vi "RSZVB Get IMOD Upper Tone Source.vi"(8 "error in (no error)":errorcluster {"code" format="%.0x"}, 10 "Channel (1)":i32=1, 11 "VISA session":refnum<visa-resource-name>) -> (0 "error out":errorcluster {"code" format="%.0x"}, 1 "Source":i32, 3 "dup VISA session":refnum<visa-resource-name>, 5 "Source Number":i32)   [LabVIEW 2011]
doc: "This VI returns the source for the upper tone signal that is used for the intermodulation measurement.\n\nNote(s):\n\n(1) This VI is not available for R&S ZVB instrument.\n\nRemote-control command(s):\n[SENSe<Ch>:]FREQuency:IMODulation:UTONe?"
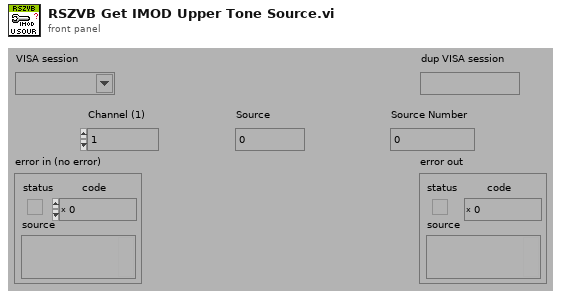
[diagram p1: front panel]
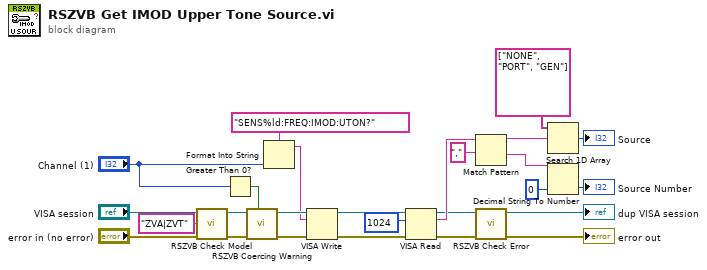
[diagram p0: block diagram]
diagram:
  n1 = call "RSZVB Check Model.vi"("error in (no error)"="error in (no error)", "Model"="ZVA|ZVT", "VISA session"="VISA session") -> ("error out"=w2:errorcluster, "dup VISA session"=w3:refnum<visa-resource-name>)  [unwired: 7 in]
  n2 = Greater Than 0?(x="Channel (1)") -> (x > 0?=w13:bool)
  n3 = call "RSZVB Coercing Warning.vi"("In Range?"=w13, "error in (no error)"=w2, "VISA session"=w3) -> ("error out"=w16:errorcluster, "dup VISA session"=w15:refnum<visa-resource-name>)  [unwired: 7 in]
  n4 = Format Into String(format string="SENS%ld:FREQ:IMOD:UTON?", "Channel (1)") -> (resulting string=w14:string)  [unwired: 2 in, 1 out]
  n5 = VISA Write(VISA resource name=w15, write buffer=w14, error in (no error)=w16) -> (VISA resource name out=w17:refnum<visa-resource-name>, error out=w18:errorcluster)  [unwired: 1 out]
  n6 = VISA Read(VISA resource name=w17, byte count=u32 1024 ("byte count (0)"), error in (no error)=w18) -> (VISA resource name out=w20:refnum<visa-resource-name>, read buffer=w26:string, error out=w21:errorcluster)  [unwired: 1 out]
  n7 = Match Pattern(string=w26, regular expression="," ("search string/char (-)")) -> (before substring=w23:string, after substring=w24:string)  [unwired: 1 in, 2 out]
  n8 = call "RSZVB Check Error.vi"("error in (no error)"=w21, "VISA session"=w20) -> ("error out"=→"error out":errorcluster, "dup VISA session"=→"dup VISA session":refnum<visa-resource-name>)  [unwired: 8 in]
  n9 = Search 1D Array(1D array=string[] ["NONE", "PORT", "GEN"], element=w23) -> (index of element=→"Source":i32)  [unwired: 1 in]
  n10 = Decimal String To Number(string=w24, default (0L)=0) -> (number=→"Source Number":i32)  [unwired: 1 in, 1 out]
